vi "SP Append Frequency Waveform.vi"(6 "Number of Points":i32, 7 "Attribute Name (NI_ChannelName)":string="NI_ChannelName", 8 "error in (no error)":errorcluster, 9 "dF":dbl, 10 "F0":dbl, 11 "Waveforms in":waveform(dbl)[](array[waveform])) -> (0 "error out":errorcluster, 3 "Waveforms out":waveform(dbl)[](array[waveform]))   [LabVIEW 2011]
uses:
  TypeDefs/SP Channel Type.ctl
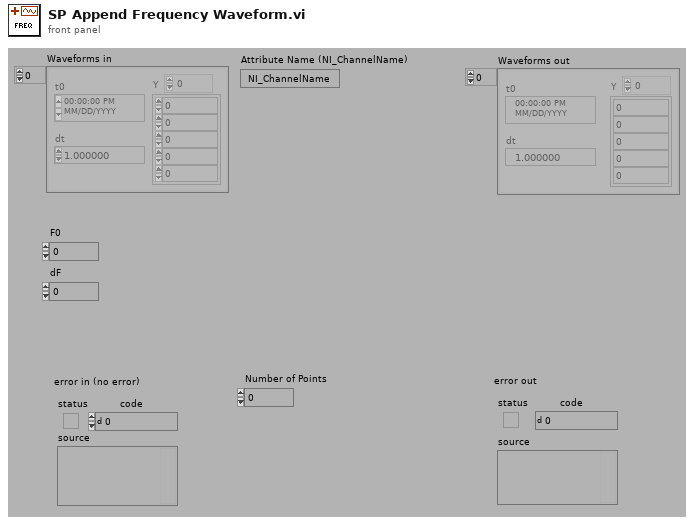
[diagram p1: front panel]
types:
  T1 = typedef "SP Channel Type.ctl" = enum16{"Frequency", "Data", "Limit", "Adapter", "Memory", "Value", "Value Limit"}
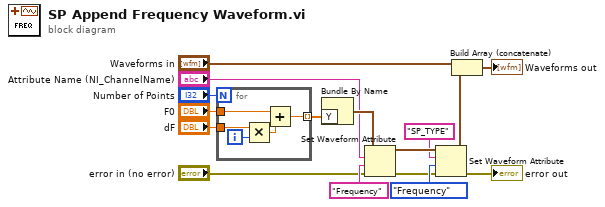
[diagram p0: block diagram]
diagram:
  n1 = for {
    N: "Number of Points" -> [_]
    tunnel: "F0" -> [w18]
    tunnel: "dF" -> [w20]
    tunnel: [w17] -> w14 mode=indexing
    i -> [w21]
    n2 = Multiply(x=w20, y=w21) -> (x*y=w19:dbl)
    n3 = Add(x=w18, y=w19) -> (x+y=w17:dbl)
  }
  n4 = Bundle By Name("Y"=w14) -> (w16:waveform(dbl))  [unwired: 1 out]
  n5 = Set Waveform Attribute(4:"error in (no error)", 5:"Frequency", 6:"Attribute Name (NI_ChannelName)", 7:w16) -> (0:w6:errorcluster, 3:w4:waveform(dbl))  [unwired: 1 out]
  n6 = Set Waveform Attribute(4:w6, 5:SP_Channel_Type."Frequency" ("Channel Type"), 6:"SP_TYPE", 7:w4) -> (0:→"error out":errorcluster, 3:w3:waveform(dbl))  [unwired: 1 out]
  n7 = Build Array (concatenate)("Waveforms in", w3) -> (→"Waveforms out":waveform(dbl)[])
